vi "Find Duplicate Test.vi"() -> (0 "error out":errorcluster, 2 "Success NO Duplicate":bool, 3 "Success Duplicate Detected":bool)   [LabVIEW 2014, in "TBM Tests.lvlib"]
doc: "Tests the Add Line and Remove Line functions."
uses:
  TBM Tests.lvlib
  module configuration/TBM module configuration.lvclass
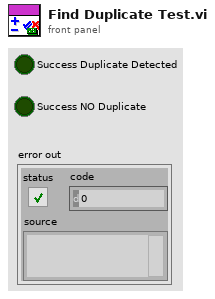
[diagram p1: front panel]
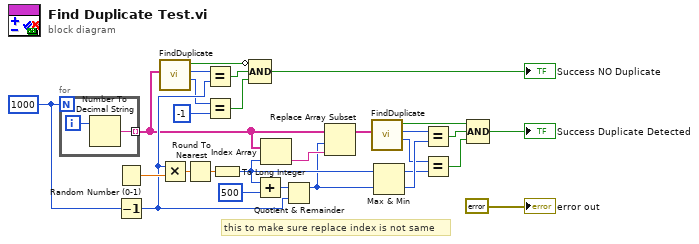
[diagram p0: block diagram]
diagram:
  w28 = 1000
  # "this to make sure replace index is not same"
  n1 = for {
    N: w28 -> [_]
    tunnel: [w29] -> w1 mode=indexing
    i -> [w30]
    n2 = Number To Decimal String(number=w30) -> (decimal integer string=w29:string)  [unwired: 1 in]
  }
  n3 = Random Number (0-1)() -> (number: 0 to 1=w27:dbl)
  n4 = Decrement(x=w28) -> (x-1=w13:i32)
  n5 = call "FindDuplicate.vi"("Array"=w1) -> ("Index 2"=w4:i32, "Index 1"=w3:i32, "Duplicate"=w2:bool)  [unwired: 8 in]
  n6 = Multiply(x=w13, y=w27) -> (x*y=w26:dbl)
  n7 = Round To Nearest(number=w26) -> (nearest integer value=w25:dbl)
  n8 = Equal?(x=w3, y=w13) -> (x = y?=w18:bool)
  n9 = Equal?(x=w4, y=-1 ("x")) -> (x = y?=w19:bool)
  n10 = To Long Integer(number=w25) -> (32bit integer=w12:i32)
  n11 = Compound Arithmetic op=AND(invert w2, w18, w19) -> (→"Success NO Duplicate":bool)
  n12 = Add(x=w12, y=500) -> (x+y=w14:i32)
  n13 = Index Array(array=w1, index=w12) -> (element=w24:string)
  n14 = Quotient & Remainder(x=w14, y=w13) -> (x-y*floor(x/y)=w11:i32)  [unwired: 1 out]
  n15 = Replace Array Subset(array=w1, new element=w24, index=w11) -> (w8:string[])
  n16 = call "FindDuplicate.vi"("Array"=w8) -> ("Index 2"=w5:i32, "Index 1"=w6:i32, "Duplicate"=w7:bool)  [unwired: 8 in]
  n17 = Max & Min(x=w12, y=w11) -> (max(x,y)=w9:i32, min(x,y)=w10:i32)
  n18 = Equal?(x=w6, y=w10) -> (x = y?=w23:bool)
  n19 = Equal?(x=w5, y=w9) -> (x = y?=w22:bool)
  n20 = Compound Arithmetic op=AND(w7, w23, w22) -> (→"Success Duplicate Detected":bool)
  "error out" <- errorcluster {"status"=FALSE, "code"=0, "source"=""} ("error out")
